vi "read-error-invalid-queues.vi"() -> (0 "Subsystem error string":string, 3 "Invalid code string":string)   [LabVIEW 2017]
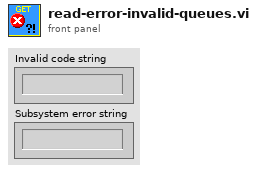
[diagram p1: front panel]
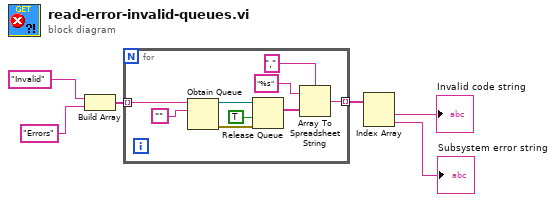
[diagram p0: block diagram]
diagram:
  n1 = Build Array("Invalid", "Errors") -> (w4:string[])
  n2 = for {
    tunnel: w4 -> [w10] mode=indexing
    tunnel: [w7] -> w3 mode=indexing
    n3 = Obtain Queue(name (unnamed)=w10, element data type="") -> (queue out=w14:refnum<queue>, error out=w13:errorcluster)  [unwired: 3 in, 1 out]
    n4 = Release Queue(queue=w14, force destroy? (F)=TRUE, error in (no error)=w13) -> (remaining elements=w8:string[])  [unwired: 2 out]
    n5 = Array To Spreadsheet String(delimiter (Tab)=",", array=w8, 3:"%s" ("format string")) -> (spreadsheet string=w7:string)
  }
  n6 = Index Array(array=w3) -> (element #1=→"Invalid code string":string, element #2=→"Subsystem error string":string)  [unwired: 2 in]
